vi "Generic command handler.vi"(8 "error in (no error)":errorcluster, 10 "Message in":refnum<class "GenericMessage.lvclass">, 11 "Galvo in":refnum<class "ImagingModeSPIM.lvclass">) -> (0 "error out":errorcluster, 2 "value":string, 3 "Galvo out":refnum<class "ImagingModeSPIM.lvclass">)   [LabVIEW 2012, in "ImagingModeSPIM.lvclass"]
doc: "The generic_command_handler processes the command 'generic'. Commands which are not part of the predefined list of commands fall under the 'generic' command for special activity."
uses:
  ImagingModeSPIM.lvclass
  <vilib>/Distrio/Murmex/GenericMessage/GenericMessage.lvclass
  <vilib>/Distrio/Murmex/Murmex/Murmex.lvclass
  <vilib>/Distrio/Murmex/Message/Add or replace parameter.vi
panel:
  # "This method is called when the GENERIC\ntrigger is sent. \n\nOverride this method when your component needs to\nrespond to this trigger. \n\nCall parent for proper implementation"
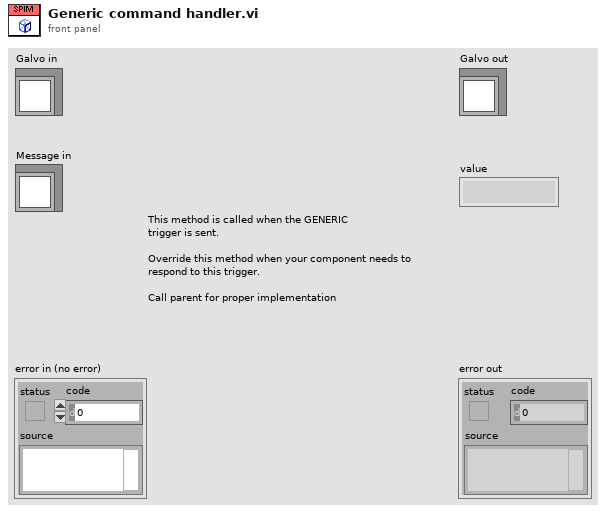
[diagram p1: front panel]
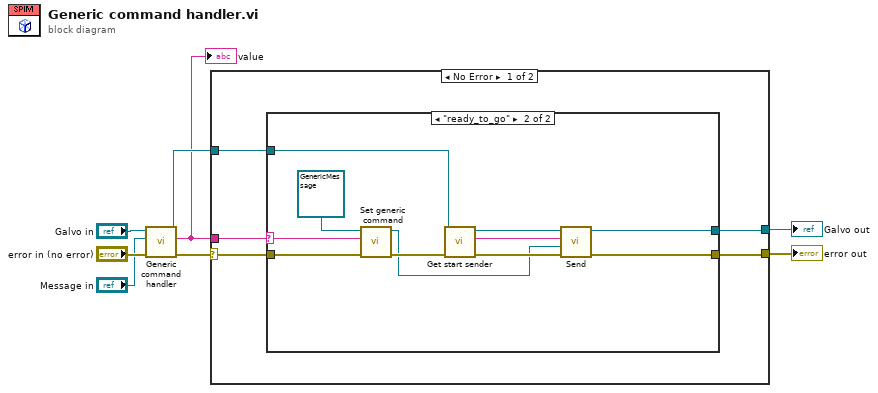
[diagram p0: block diagram]
diagram:
  n1 = call-parent "Generic command handler.vi"("error in (no error)"="error in (no error)", "Message in"="Message in", "Murmex in"="Galvo in") -> ("error out"=w6:errorcluster, "value"=w1:string, "Murmex out"=w5:refnum<class "ImagingModeSPIM.lvclass">)  [unwired: 6 in]
  "value" <- w1
  n2 = case shown="No Error" w6 {
    selector: w6 -> [w9 w27]
    tunnel: w5 -> [w12 w28]
    tunnel: [w10 w27] -> w3
    tunnel: [w11 w28] -> w2
    tunnel: w1 -> [w13 _]
    frame No Error {
      n3 = case shown="\"ready_to_go\"" w13 {
        selector: w13 -> [_ w24]
        tunnel: w12 -> [w15 w26]
        tunnel: [w15 w18] -> w11
        tunnel: [w14 w20] -> w10
        tunnel: w9 -> [w14 w25]
        frame Default {
        }
        frame "ready_to_go" {
          n4 = call <vilib>:"Set generic command.vi"("error in (no error)"=w25, "generic command"=w24, "GenericMessage in"=refnum<class "GenericMessage.lvclass"> refnum ("Distrio Murmex 1.2:GenericMessage")) -> ("error out"=w22:errorcluster, "GenericMessage out"=w16:refnum<class "GenericMessage.lvclass">)  [unwired: 7 in]
          n5 = call-dynamic "Get start sender.vi"("error in (no error)"=w22, "ImagingModeSPIM in"=w26) -> ("error out"=w21:errorcluster, "start sender"=w17:string, "ImagingModeSPIM out"=w19:refnum<class "ImagingModeSPIM.lvclass">)  [unwired: 7 in]
          n6 = call <vilib>:"Send.vi"("error in (no error)"=w21, "Message"=w16, "recipient"=w17, "Murmex in"=w19) -> ("error out"=w20:errorcluster, "Murmex out"=w18:refnum<class "ImagingModeSPIM.lvclass">)  [unwired: 6 in]
        }
      }
    }
    frame Error {
    }
  }
  "error out" <- w3
  "Galvo out" <- w2
